vi "toDevBoolean.vi"(1 "ArgIO":cluster{"num data":u8[], "str data":string[]}) -> (0 "argout":bool=TRUE)   [LabVIEW 2014, in "tango.lvlib"]
uses:
  tango.lvlib
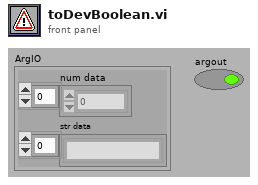
[diagram p1: front panel]
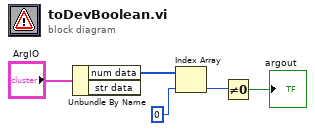
[diagram p0: block diagram]
diagram:
  n1 = Unbundle By Name("ArgIO") -> ("num data"=w2:u8[])  [unwired: 1 out]
  n2 = Index Array(array=w2, index=0 ("indice")) -> (element=w1:u8)
  n3 = Not Equal To 0?(x=w1) -> (x != 0?=→"argout":bool)
